vi "Pack PII Error_1SDI_v00.vi"(8 "PII+Error HD B":T5, 9 "PII+Error HD A":T5, 11 "PII+Error EPR BS":T8) -> (0 "Theta":T2, 1 "Thresholds":cluster{"Lock":T4, "Re-Scan":T4}, 3 "Error packed":T3={"Pre-Offset"={"Pre-Offset 1"=2, "Pre-Offset 2"=0, "Pre-Offset 3"=0, "Pre-Offset 4"=0, "Pre-Offset 5"=2}, "Post-Offset "={"Offset 1"=0, "Offset 2"=0, "Offset 3"=0, "Offset 4"=0, "Offset 5"=0}, "Gains"={"Gain 1"=0, "Gain 2"=0, "Gain 3"=0, "Gain 4"=0, "Gain 5"=0}, "Bit Shifts"={"Bit Shift 1"=0, "Bit Shift 2"=300, "Bit Shift 3"=0, "Bit Shift 4"=0, "Bit Shift 5"=0}})   [LabVIEW 2011]
doc: "Packages individual values related to error signal scaling from the user interface into data structures compatible with FPGA_Cavities.VI\n(very messy, could use a tidy)."
uses:
  Strict Type Defs/1SDI Errors I16.ctl
  Strict Type Defs/Error Scale 1SDI.ctl
  Strict Type Defs/PII and Error Graph.ctl
  Strict Type Defs/Errors Converted Graph.ctl
  Strict Type Defs/PII individual.ctl
  Strict Type Defs/PII and Error Graph HD.ctl
  Strict Type Defs/Errors Converted Graph HD.ctl
  Strict Type Defs/Lock Thresh 1SDI.ctl
  Strict Type Defs/Theta graph.ctl
panel:
  in  "Bit Shifts":T1
  in  "Theta typedef":T2
  in  "Error scale graph type":T3={"Pre-Offset"={"Pre-Offset 1"=2, "Pre-Offset 2"=0, "Pre-Offset 3"=0, "Pre-Offset 4"=0, "Pre-Offset 5"=2}, "Post-Offset "={"Offset 1"=0, "Offset 2"=300, "Offset 3"=0, "Offset 4"=0, "Offset 5"=0}, "Gains"={"Gain 1"=0, "Gain 2"=300, "Gain 3"=0, "Gain 4"=0, "Gain 5"=0}, "Bit Shifts"={"Bit Shift 1"=0, "Bit Shift 2"=300, "Bit Shift 3"=0, "Bit Shift 4"=0, "Bit Shift 5"=0}}
  in  "Thresholds type def":cluster{"Lock":T4, "Re-Scan":T4}
  in  "Re-Scan Thresh":T4
  in  "Lock Thresh":T4
  in  "Pre Offset":T1
  in  "Offset":T1
  in  "Gains":T1
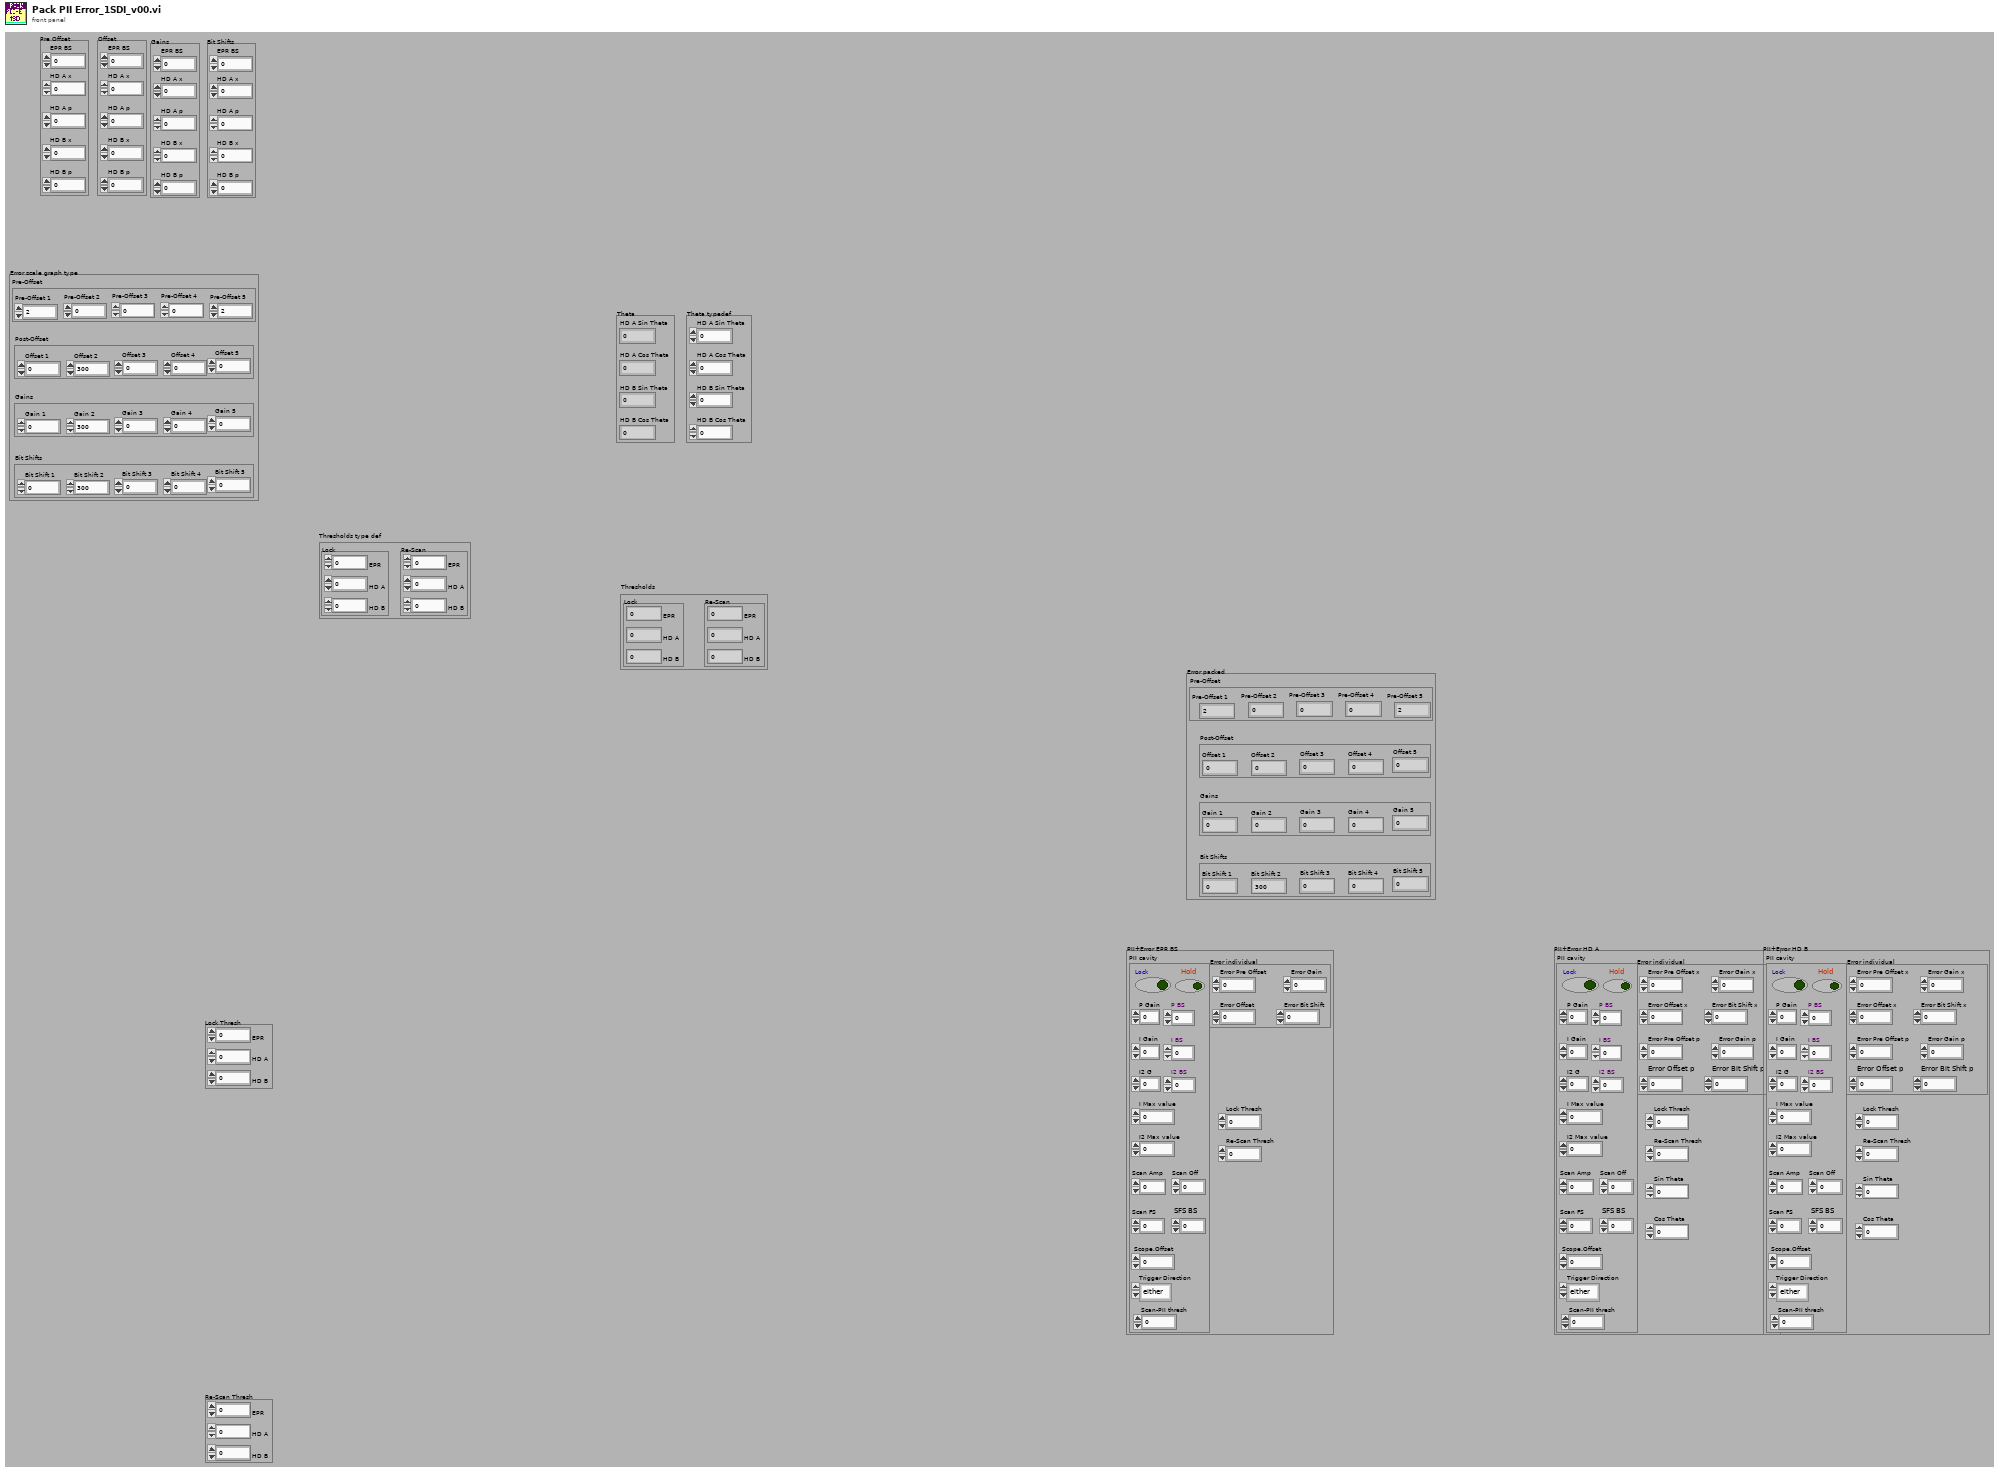
[diagram p1: front panel]
types:
  T1 = typedef "1SDI Errors I16.ctl" = cluster{"EPR BS":i16, "HD A x":i16, "HD A p":i16, "HD B x":i16, "HD B p":i16}
  T2 = typedef "Theta graph.ctl" = cluster{"HD A Sin Theta":i32, "HD A Cos Theta":i32, "HD B Sin Theta":i32, "HD B Cos Theta":i32}
  T3 = typedef "Error Scale 1SDI.ctl" = cluster{"Pre-Offset":cluster{"Pre-Offset 1":i16, "Pre-Offset 2":i16, "Pre-Offset 3":i16, "Pre-Offset 4":i16, "Pre-Offset 5":i16}, "Post-Offset ":cluster{"Offset 1":i16, "Offset 2":i16, "Offset 3":i16, "Offset 4":i16, "Offset 5":i16}, "Gains":cluster{"Gain 1":i16, "Gain 2":i16, "Gain 3":i16, "Gain 4":i16, "Gain 5":i16}, "Bit Shifts":cluster{"Bit Shift 1":i16, "Bit Shift 2":i16, "Bit Shift 3":i16, "Bit Shift 4":i16, "Bit Shift 5":i16}}
  T4 = typedef "Lock Thresh 1SDI.ctl" = cluster{"EPR":i16, "HD A":i16, "HD B":i16}
  T5 = typedef "PII and Error Graph HD.ctl" = cluster{"Error individual":T6, "PII cavity":T7, "Lock Thresh":i16, "Re-Scan Thresh":i16, "Sin Theta":i32, "Cos Theta":i32}
  T6 = typedef "Errors Converted Graph HD.ctl" = cluster{"Error Pre Offset x":i16, "Error Offset x":i16, "Error Gain x":i16, "Error Bit Shift x":i16, "Error Pre Offset p":i16, "Error Offset p":i16, "Error Gain p":i16, "Error Bit Shift p":i16}
  T7 = typedef "PII individual.ctl" = cluster{"Lock":bool, "Hold":bool, "P Gain":i32, "P BS":i16, "I Gain":i32, "I BS":i16, "I2 G":i32, "I2 BS":i16, "Scan Amp":i16, "Scan Off":i16, "Scan FS":u16, "SFS BS":i16, "I Max value":i32, "I2 Max value":i32, "Scope.Offset":i16, "Trigger Direction":enum8{"either", "minus-plus", "plus-minus"}, "Scan-PII thresh":i16}
  T8 = typedef "PII and Error Graph.ctl" = cluster{"Error individual":T9, "PII cavity":T7, "Lock Thresh":i16, "Re-Scan Thresh":i16}
  T9 = typedef "Errors Converted Graph.ctl" = cluster{"Error Pre Offset":i16, "Error Offset":i16, "Error Gain":i16, "Error Bit Shift":i16}
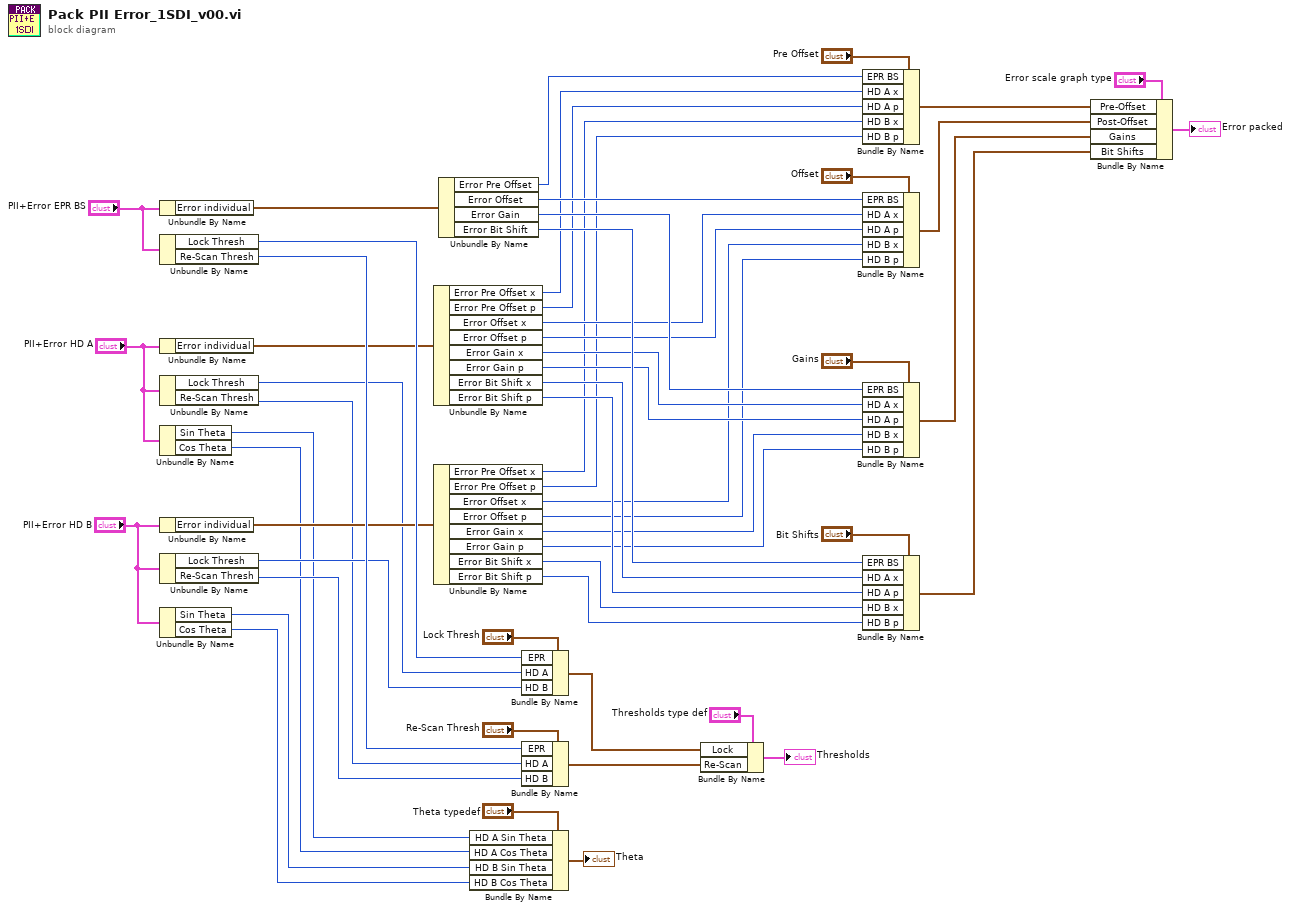
[diagram p0: block diagram]
diagram:
  n1 = Unbundle By Name("PII+Error EPR BS") -> ("Error individual"=w53:T9)
  n2 = Unbundle By Name("PII+Error EPR BS") -> ("Lock Thresh"=w45:i16, "Re-Scan Thresh"=w43:i16)
  n3 = Unbundle By Name("PII+Error HD A") -> ("Error individual"=w32:T6)
  n4 = Unbundle By Name("PII+Error HD A") -> ("Lock Thresh"=w14:i16, "Re-Scan Thresh"=w12:i16)
  n5 = Unbundle By Name("PII+Error HD A") -> ("Sin Theta"=w9:i32, "Cos Theta"=w8:i32)
  n6 = Unbundle By Name("PII+Error HD B") -> ("Error individual"=w23:T6)
  n7 = Unbundle By Name("PII+Error HD B") -> ("Lock Thresh"=w13:i16, "Re-Scan Thresh"=w11:i16)
  n8 = Unbundle By Name("PII+Error HD B") -> ("Sin Theta"=w6:i32, "Cos Theta"=w5:i32)
  n9 = Unbundle By Name(w32) -> ("Error Pre Offset x"=w31:i16, "Error Pre Offset p"=w30:i16, "Error Offset x"=w29:i16, "Error Offset p"=w28:i16, "Error Gain x"=w27:i16, "Error Gain p"=w26:i16, "Error Bit Shift x"=w25:i16, "Error Bit Shift p"=w24:i16)
  n10 = Unbundle By Name(w23) -> ("Error Pre Offset x"=w15:i16, "Error Pre Offset p"=w16:i16, "Error Offset x"=w17:i16, "Error Offset p"=w18:i16, "Error Gain x"=w19:i16, "Error Gain p"=w20:i16, "Error Bit Shift x"=w21:i16, "Error Bit Shift p"=w22:i16)
  n11 = Unbundle By Name(w53) -> ("Error Pre Offset"=w52:i16, "Error Offset"=w51:i16, "Error Gain"=w50:i16, "Error Bit Shift"=w33:i16)
  n12 = Bundle By Name(cluster="Theta typedef", "HD A Sin Theta"=w9, "HD A Cos Theta"=w8, "HD B Sin Theta"=w6, "HD B Cos Theta"=w5) -> (→"Theta":T2)
  n13 = Bundle By Name(cluster="Lock Thresh", "EPR"=w45, "HD A"=w14, "HD B"=w13) -> (w41:T4)
  n14 = Bundle By Name(cluster="Re-Scan Thresh", "EPR"=w43, "HD A"=w12, "HD B"=w11) -> (w40:T4)
  n15 = Bundle By Name(cluster="Thresholds type def", "Lock"=w41, "Re-Scan"=w40) -> (→"Thresholds":cluster{"Lock":T4, "Re-Scan":T4})
  n16 = Bundle By Name(cluster="Pre Offset", "EPR BS"=w52, "HD A x"=w31, "HD A p"=w30, "HD B x"=w15, "HD B p"=w16) -> (w4:T1)
  n17 = Bundle By Name(cluster="Offset", "EPR BS"=w51, "HD A x"=w29, "HD A p"=w28, "HD B x"=w17, "HD B p"=w18) -> (w3:T1)
  n18 = Bundle By Name(cluster="Gains", "EPR BS"=w50, "HD A x"=w27, "HD A p"=w26, "HD B x"=w19, "HD B p"=w20) -> (w2:T1)
  n19 = Bundle By Name(cluster="Bit Shifts", "EPR BS"=w33, "HD A x"=w25, "HD A p"=w24, "HD B x"=w21, "HD B p"=w22) -> (w1:T1)
  n20 = Bundle By Name(cluster="Error scale graph type", "Pre-Offset"=w4, "Post-Offset"=w3, "Gains"=w2, "Bit Shifts"=w1) -> (→"Error packed":T3)
